vi "PrintDebugInfo.vi"(8 "error in (no error)":errorcluster, 11 "CDependencyInspector in":refnum<class "CDependencyInspection.lvclass">) -> (0 "error out":errorcluster, 1 "Debug string":string, 3 "CDependencyInspector out":refnum<class "CDependencyInspection.lvclass">)   [LabVIEW 2020, in "DependencyInspection.lvlib" / "CDependencyInspection.lvclass"]
uses:
  CDependencyInspection.lvclass
  CDependencyInspection.lvclass/CDependencyInspection.ctl
  CDebugInfo/CDebugInfo.lvclass
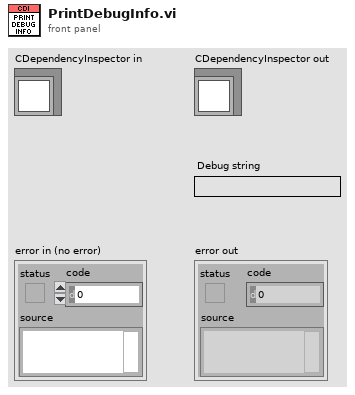
[diagram p1: front panel]
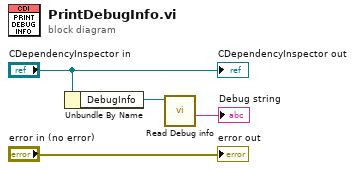
[diagram p0: block diagram]
diagram:
  n1 = Unbundle By Name("CDependencyInspector in") -> ("DebugInfo"=w2:refnum<class "CDebugInfo.lvclass">)
  n2 = call-dynamic "Read Debug info.vi"("CDebugInfo in"=w2) -> ("Debug info"=→"Debug string":string)  [unwired: 9 in, 1 out]
  "error out" <- "error in (no error)"
  "CDependencyInspector out" <- "CDependencyInspector in"
